vi "RetrieveAcPwrMeasurementData.vi"(0 "WaveformChartReference":refnum<vi>, 1 "PlotYScale":u32[](array[numeric]), 5 "WaveformArrayIn":waveform(dbl)[](array[waveform]), 11 "error in (no error)":errorcluster) -> (4 "WaveformArrayOut":waveform(dbl)[](array[waveform]), 6 "OutputString(Chroma)":string, 8 "Incorrect DataType?":bool, 10 "Status Byte Register(NHRRGS)":T1(array[cluster]), 15 "error out":errorcluster)   [LabVIEW 2018, in "AcPwrShared.lvlib"]
doc: "This VI takes in the measurement data from an AcPwr Plugin and retrieves additional information from the attributes defined in the AcPwrAttriutesTypeDef.ctl such as Register Status Byte."
uses:
  AcPwrShared/AcPwrShared.lvlib
  AcPwrShared/clAcPwrAttributes.ctl
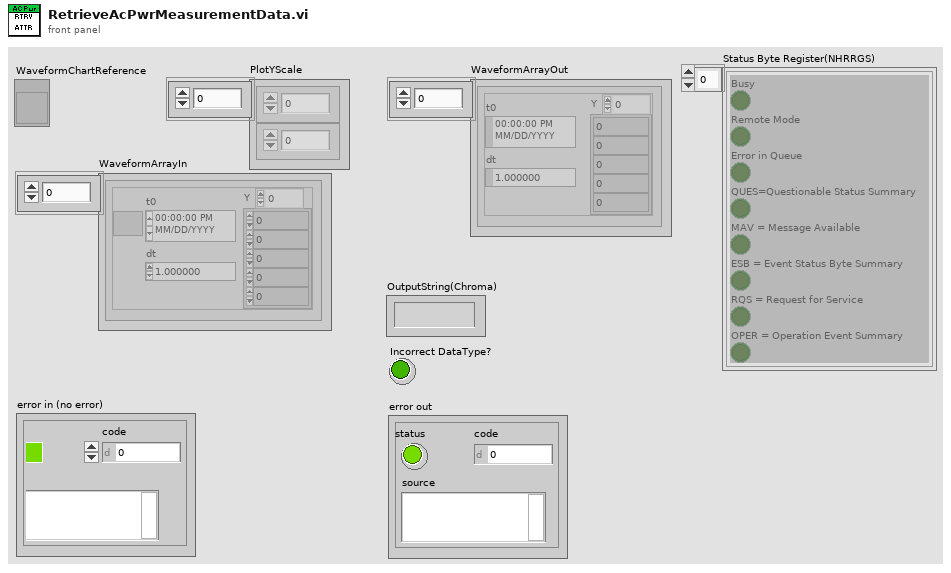
[diagram p1: front panel]
types:
  T1 = cluster{"Busy":bool, "Remote Mode":bool, "Error in Queue":bool, "QUES=Questionable Status Summary":bool, "MAV = Message Available":bool, "ESB = Event Status Byte Summary":bool, "RQS = Request for Service":bool, "OPER = Operation Event Summary":bool}[]
  T2 = typedef "AcPwrShared.lvlib/clAcPwrAttributes.ctl" = cluster{"ProtectionStatusString":string, "Handle_MeasurementType":string, "Status Byte Register":cluster{"Busy":bool, "Remote Mode":bool, "Error in Queue":bool, "QUES=Questionable Status Summary":bool, "MAV = Message Available":bool, "ESB = Event Status Byte Summary":bool, "RQS = Request for Service":bool, "OPER = Operation Event Summary":bool}}
  T3 = cluster{"Busy":bool, "Remote Mode":bool, "Error in Queue":bool, "QUES=Questionable Status Summary":bool, "MAV = Message Available":bool, "ESB = Event Status Byte Summary":bool, "RQS = Request for Service":bool, "OPER = Operation Event Summary":bool}
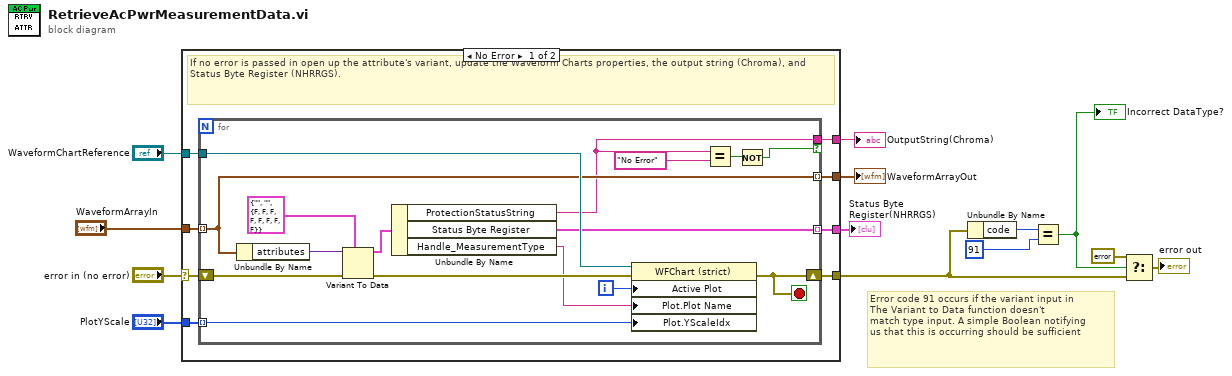
[diagram p0: block diagram]
diagram:
  # "Error code 91 occurs if the variant input in \nThe Variant to Data function doesn't \nmatch type input. A simple Boolean notifying \nus that this is occurring should be sufficient"
  n1 = case shown="No Error" "error in (no error)" {
    selector: "error in (no error)" -> [w21 w38]
    tunnel: [w20 w38] -> w4
    tunnel: [w19 _] -> w3
    tunnel: "WaveformChartReference" -> [w16 _]
    tunnel: "PlotYScale" -> [w18 _]
    tunnel: [w17 _] -> w10
    tunnel: "WaveformArrayIn" -> [w15 _]
    tunnel: [w14 _] -> w1
    frame No Error {
      # "If no error is passed in open up the attribute's variant, update the Waveform Charts properties, the output string (Chroma), and Status Byte Register (NHRRGS)."
      n2 = for {
        shift-right: [w34] -> w20
        shift-left: w21 -> [w29]
        tunnel: [w31] -> w19 mode=indexing
        tunnel: w16 -> [w36]
        tunnel: w18 -> [w35] mode=indexing
        tunnel: [w24] -> w17 if=w27
        tunnel: w15 -> [w31] mode=indexing
        tunnel: [w22] -> w14 mode=indexing
        i -> [w37]
        stop <- w34 stop-if-true
        n3 = Unbundle By Name(w31) -> ("attributes"=w30:variant)
        n4 = Variant To Data(error in=w29, type=T2 {"ProtectionStatusString"="", "Handle_MeasurementType"="", "Status Byte Register"={"Busy"=FALSE, "Remote Mode"=FALSE, "Error in Queue"=FALSE, "QUES=Questionable Status Summary"=FALSE, "MAV = Message Available"=FALSE, "ESB = Event Status Byte Summary"=FALSE, "RQS = Request for Service"=FALSE, "OPER = Operation Event Summary"=FALSE}} ("Attributes"), Variant=w30) -> (data=w25:T2, error out=w28:errorcluster)
        n5 = Unbundle By Name(w25) -> ("ProtectionStatusString"=w24:string, "Status Byte Register"=w22:T3, "Handle_MeasurementType"=w23:string)
        n6 = property on="Property Node" class="WFChart (strict)"(reference=w36, error in=w28, "Active Plot"=w37, "Plot.Plot Name"=w23, "Plot.YScaleIdx"=w35) -> (error out=w34:errorcluster)  [unwired: 1 out]
        n7 = Equal?(x=w24, y="No Error") -> (x = y?=w33:bool)
        n8 = Not(x=w33) -> (.not. x?=w27:bool)
      }
    }
    frame Error {
    }
  }
  "OutputString(Chroma)" <- w10
  "WaveformArrayOut" <- w3
  "Status Byte Register(NHRRGS)" <- w1
  n9 = Unbundle By Name(w4) -> ("code"=w9:i32)
  n10 = Equal?(x=w9, y=91) -> (x = y?=w7:bool)
  "Incorrect DataType?" <- w7
  n11 = Select(t=errorcluster {"status"=FALSE, "code"=0, "source"=""} ("error IO"), s=w7, f=w4) -> (s? t:f=→"error out":errorcluster)
